vi "VIinClass.vi"(10 "Y":dbl, 11 "X":dbl) -> (3 "Result":dbl)   [LabVIEW 2023, in "ClassForClassMemberCall.lvclass"]
uses:
  ClassForClassMemberCall.lvclass
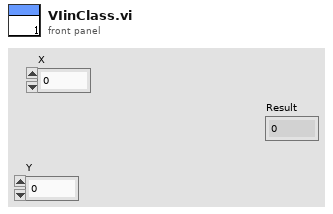
[diagram p1: front panel]
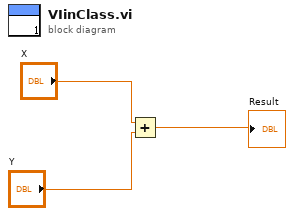
[diagram p0: block diagram]
diagram:
  n1 = Add(x="X", y="Y") -> (x+y=→"Result":dbl)
